vi "Test_RegisterForWrongType_MCListbox_Error.vi"(8 "error in (no error)":errorcluster, 11 "TestActorEvents In":refnum<class "TestActorEvents.lvclass">) -> (0 "error out":errorcluster, 3 "TestActorEvents Out":refnum<class "TestActorEvents.lvclass">)   [LabVIEW 2017, in "TestActorEvents.lvlib" / "TestActorEvents.lvclass"]
uses:
  TestActorEvents.lvclass
  Source/Framework/IViewModel/IViewModel/IViewModel.lvclass
  C:/Git/mva-framework/Source/Framework/IObserver/IObserver/IObserver.lvclass
  C:/Git/mva-framework/Source/Framework/IViewManager/IViewManager/IViewManager.lvclass
  C:/Program Files (x86)/National Instruments/LabVIEW 2017/vi.lib/ActorFramework/Actor/Actor.lvclass
  ViewableMCListboxBadReg/ViewableMCListboxBadReg.lvclass
  C:/Git/mva-framework/Test/Doubles/ViewableDoubles/LeakyViewable/LeakyViewable.lvclass
  C:/Git/mva-framework/Source/Framework/IViewable/IViewable/IViewable.lvclass
  Source/Framework/IModel/IModel/IModel.lvclass
  Source/Framework/Mediator/Mediator/Mediator.lvclass
  C:/Git/mva-framework/Source/Framework/IMediator/IMediator/IMediator.lvclass
  Doubles/ViewableDoubles/LeakyViewable/Leak Location.ctl
  Doubles/ViewableDoubles/LeakyViewable/LeakyViewable.lvclass/LeakyViewable.ctl
  gpm_packages/@cs/event-logger/Source/Composed Log/LoggerReference/LoggerReference.lvclass/LoggerReference.ctl
  Source/Framework/IObserver/IObserver/IObserver.lvclass/IObserver.ctl
  Source/Framework/IMediator/IMediator/IMediator.lvclass/IMediator.ctl
  Source/Framework/IViewModel/IViewModel/IViewModel.lvclass/IViewModel.ctl
  Source/Framework/IViewManager/IViewManager Messages/Launch Nested Views Msg/Launch Nested Views Msg.lvclass/Launch Nested Views Msg.ctl
  Source/Framework/IViewManager/IViewManager/IViewManager.lvclass/IViewManager.ctl
  <vilib>/ActorFramework/Message Enqueuer/Message Enqueuer.lvclass/Message Enqueuer.ctl
  42a2a2f1-017f-46ad-b297-243c6642a3b4.vi
  42a2a2f1-017f-46ad-b297-243c6642a3b4.vi/c661b006-0968-4628-b95c-c58973ad7297.vi
  Source/Framework/IObserver/IObserver/Configure Observer Logging.vi
  Source/Framework/IViewModel/IViewModel/Write Startup Model-View Configuration.vi
  Source/Framework/IMediator/IMediator/Configure Mediator.vi
  <vilib>/ActorFramework/Message Enqueuer/Enqueue.vi
  gpm_packages/@cs/event-logger/Source/Composed Log/LoggerReference/Return Aggregate Queues.vi
  gpm_packages/@cs/event-logger/Source/Composed Log/LoggerReference/Add Aggregate Log.vi
  42a2a2f1-017f-46ad-b297-243c6642a3b4.vi/c661b006-0968-4628-b95c-c58973ad7297.vi/874536e9-dd21-421b-9c6e-9da045bfbaad.vi
  Source/Framework/IViewManager/IViewManager Messages/Launch Nested Views Msg/Pack Launch Nested Views Msg.vi
  Source/Framework/IViewManager/IViewManager/Write Startup Launch Nested Views Msg.vi
  gpm_packages/@cs/event-logger/Source/Composed Log/LoggerReference/Send Add Sink.vi
  gpm_packages/@cs/event-logger/Source/Text File Sink/Text File Sink.lvclass
  C:/Git/mva-framework/gpm_packages/@cs/event-logger/Source/Composed Log/Log Sink/Log Sink.lvclass
  <vilib>/ActorFramework/Stop Msg/Stop Msg.lvclass
  C:/Program Files (x86)/National Instruments/LabVIEW 2017/vi.lib/ActorFramework/Message/Message.lvclass
  gpm_packages/@cs/event-logger/Source/Composed Log/Application Logger/Launch Worker Loop.vi
  gpm_packages/@cs/event-logger/Source/Composed Log/LoggerReference/Initialize Logger Instance.vi
  <vilib>/ActorFramework/Message Priority Queue/Priority Enqueue.vi
  Source/Framework/IViewable/IViewable/IViewable.lvclass
  gpm_packages/@cs/event-logger/Source/Composed Log/LoggerReference/LoggerReference.lvclass
  Source/Framework/IMediator/IMediatorBusMonitor/IMediatorBusMonitor.lvclass
  gpm_packages/@cs/event-logger/Source/Composed Log/IErrorFormat/IErrorFormat.lvclass
  gpm_packages/@cs/event-logger/Source/Composed Log/Log Sink/Log Sink.lvclass
  Source/Framework/IViewable/IApplicationStyle/IApplicationStyle.lvclass
  Source/Framework/IViewManager/IViewManager Messages/Launch Nested Views Msg/Launch Nested Views Msg.lvclass
  <vilib>/addons/_JKI Toolkits/VI Tester/TestCase.llb/TestCase.lvclass
  <vilib>/ActorFramework/Actor/Actor.lvclass
  Doubles/ViewableDoubles/LeakyViewable/LeakyViewable.lvclass
  C:/Program Files (x86)/National Instruments/LabVIEW 2017/vi.lib/addons/_JKI Toolkits/VI Tester/TestCase.llb/TestCase.lvclass
panel:
  out "Error Status":errorcluster
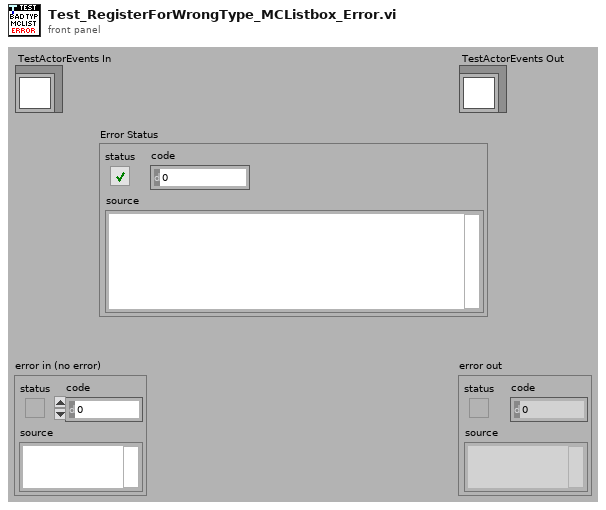
[diagram p1: front panel]
types:
  T1 = typedef "ViewableDoubles.lvlib/LeakyViewable.lvclass/Leak Location.ctl" = enum16{"Pre Launch Init", "Entering Actor Core", "Actor Core", "Exiting Actor Core", "Stop Core", "Handle Error"}
  T2 = cluster{"Location":T1, "State":refnum<class "IViewable.lvclass">, "Error Status":errorcluster}
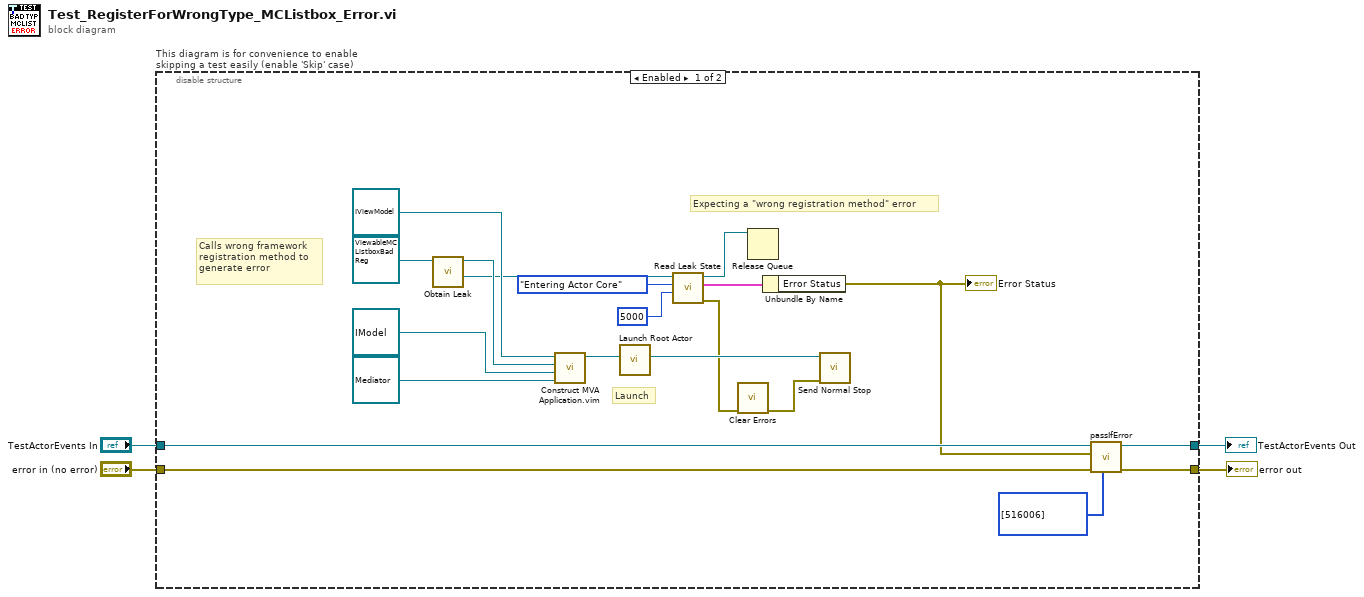
[diagram p0: block diagram]
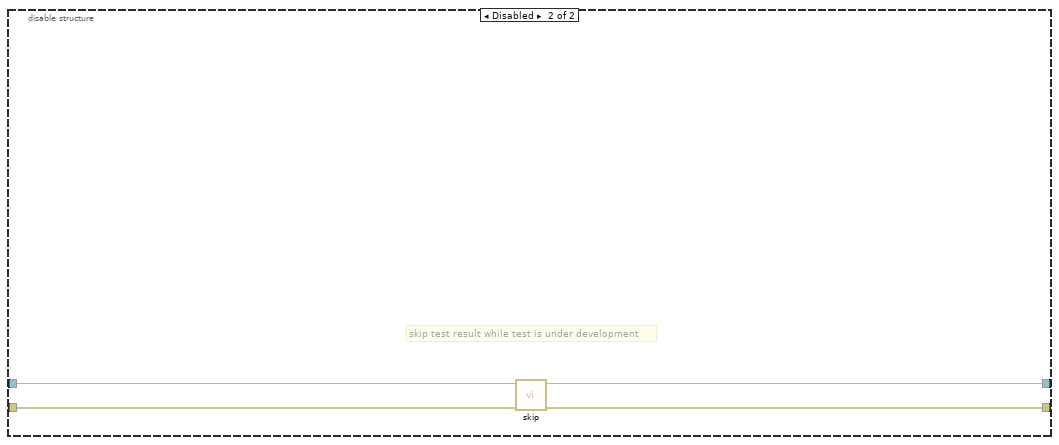
[diagram p2: hidden frame]
diagram:
  n1 = disable-structure "This diagram is for convenience to enable skipping a test easily (enable 'Skip' case)" shown="Enabled" {
    disable-tunnel: "TestActorEvents In" -> [w24 w28]
    disable-tunnel: [w23 w26] -> w1
    disable-tunnel: [w22 w27] -> w3
    disable-tunnel: "error in (no error)" -> [w21 w25]
    frame Enabled {
      # "Expecting a \"wrong registration method\" error"
      # "Calls wrong framework\nregistration method to\ngenerate error"
      # "Launch"
      n2 = call "Obtain Leak.vi"("LeakyViewable In"=refnum<class "ViewableMCListboxBadReg.lvclass"> refnum ("Startup View Configuration")) -> ("Viewable Leak Queue"=w13:refnum<queue>, "LeakyViewable Out"=w14:refnum<class "ViewableMCListboxBadReg.lvclass">)  [unwired: 9 in]
      n3 = call "Construct MVA Application.vim"("Mediator Type"=refnum<class "Mediator.lvclass"> refnum ("Mediator"), "Model Type"=refnum<class "IModel.lvclass"> refnum ("Model"), "Startup View Configuration"=w14, "IViewModel In"=refnum<class "IViewModel.lvclass"> refnum) -> ("IViewModel Out"=w16:refnum<class "IViewModel.lvclass">)  [unwired: 7 in]
      n4 = call <vilib>:"Launch Root Actor.vi"("Actor"=w16) -> ("Actor's Enqueuer"=w8:refnum<class "Message Enqueuer.lvclass">)  [unwired: 9 in, 1 out]
      n5 = call "Read Leak State.vi"("timeout in ms (-1)"=5000, "Leak Location"=Leak_Location."Entering Actor Core", "Viewable Leak Queue In"=w13) -> ("error out"=w7:errorcluster, "State Snapshot"=w10:T2, "Viewable Leak Queue"=w5:refnum<queue>)  [unwired: 5 in, 1 out]
      n6 = call <vilib>:"Clear Errors.vi"("error in (no error)"=w7) -> ("error out"=w6:errorcluster)  [unwired: 5 in, 1 out]
      n7 = Release Queue(queue=w5) -> ()  [unwired: 2 in, 3 out]
      n8 = Unbundle By Name(w10) -> ("Error Status"=w9:errorcluster)
      "Error Status" <- w9
      n9 = call <vilib>:"Send Normal Stop.vi"("error in (no error)"=w6, "Message Enqueuer"=w8) -> ()  [unwired: 9 in, 1 out]
      n10 = call-dynamic "passIfError.vi"("passing error codes (default = any error code)"=i32[] [516006], "error in (no error)"=w21, "error"=w9, "TestCase in"=w24) -> ("error out"=w22:errorcluster, "TestCase out"=w23:refnum<class "TestActorEvents.lvclass">)  [unwired: 6 in]
    }
    frame Disabled {
      # "skip test result while test is under development"
      n11 = call <vilib>:"skip.vi"("error in (no error)"=w25, "TestCase in"=w28) -> ("error out"=w27:errorcluster, "TestCase out"=w26:refnum<class "TestActorEvents.lvclass">)  [unwired: 8 in]
    }
  }
  "error out" <- w3
  "TestActorEvents Out" <- w1
